vi "Core Action.vi"(8 "error in (no error)":errorcluster, 10 "SECS-II Class":refnum<class "SECS-II Class.lvclass">, 11 "24-Host Accepts On-Line Request from Equipment in":refnum<class "24-Host Accepts On-Line Request from Equipment.lvclass">) -> (0 "error out":errorcluster, 2 "SECS-II Class Out":refnum<class "SECS-II Class.lvclass">, 3 "24-Host Accepts On-Line Request from Equipment out":refnum<class "24-Host Accepts On-Line Request from Equipment.lvclass">)   [LabVIEW 2020, in "SECS Scenarios.lvlib" / "24-Host Accepts On-Line Request from Equipment.lvclass"]
uses:
  24-Host Accepts On-Line Request from Equipment.lvclass
  D:/Dropbox/SECS/SECS_GEM v1.1.0/Com/SECS Scenarios/Scenarios Class/Scenarios Class.lvclass
  SECS Communication/SECS-II Class/SECS-II Class.lvclass
  24-Host Accepts On-Line Request from Equipment.lvclass/24-Host Accepts On-Line Request from Equipment.ctl
  SECS Communication/S1 Message Class/S1 Message Class.lvclass
  D:/Dropbox/SECS/SECS_GEM v1.1.0/Com/SECS Communication/SECS-II Class/SECS-II Class.lvclass
  Scenarios Class/Scenarios Class.lvclass/Scenarios Class.ctl
  SECS Communication/SECS-II Class/SECS-II Class.lvclass/SECS-II Class.ctl
  Scenarios Class/Reply State.ctl
  SECS Communication/SECS-II Class/Read Function.vi
  Scenarios Class/Write Reply State.vi
  Scenarios Class/Read HSMS Class.vi
  SECS Communication/HSMS Class/HSMS Class.lvclass
  Scenarios Class/Scenarios Class.lvclass
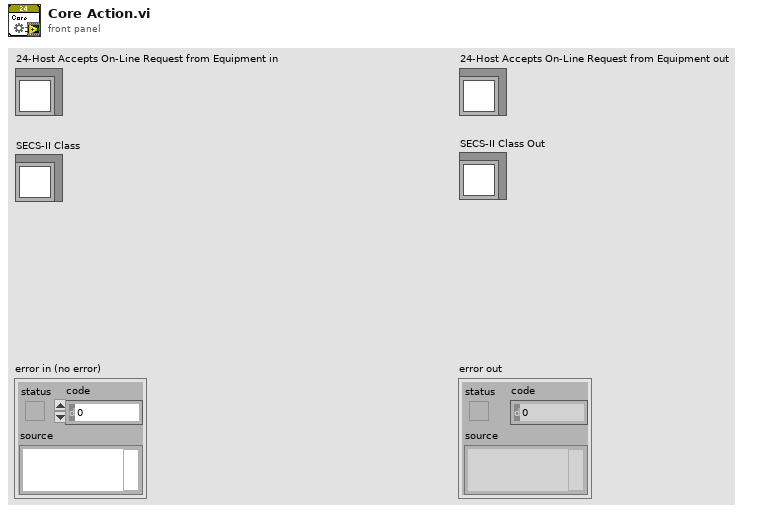
[diagram p1: front panel]
types:
  T1 = typedef "SECS Scenarios.lvlib/Scenarios Class.lvclass/Reply State.ctl" = enum16{"OK", "Illegal Data", "Unknown Stream", "Unknown Function", "Off-Line", "T3 Timeout", "Inner-Timeout"}
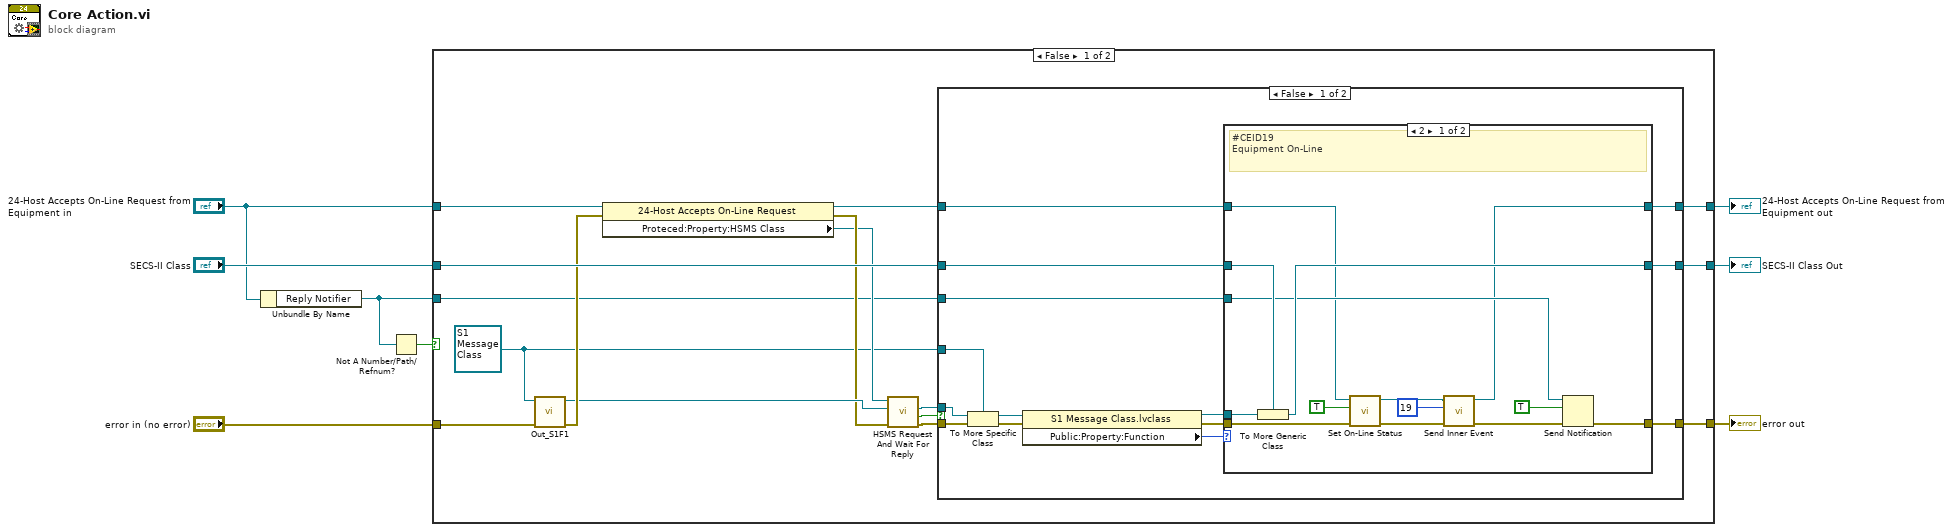
[diagram p0: block diagram]
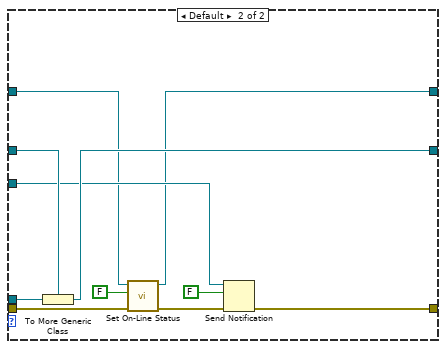
[diagram p2: hidden frame]
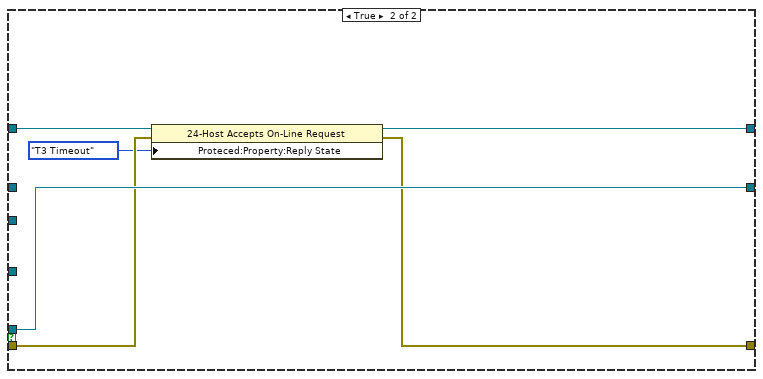
[diagram p3: hidden frame]
diagram:
  n1 = Unbundle By Name("24-Host Accepts On-Line Request from Equipment in") -> ("Reply Notifier"=w2:refnum<notifier>)
  n2 = Not A Number/Path/Refnum?(number/path/refnum=w2) -> (NaN/Path/Refnum?=w1:bool)
  n3 = case shown="False" w1 {
    tunnel: "error in (no error)" -> [w24 w72]
    tunnel: [w23 w70] -> w7
    tunnel: [w22 w72] -> w6
    tunnel: "SECS-II Class" -> [w21 w71]
    tunnel: [w20 w71] -> w4
    tunnel: "24-Host Accepts On-Line Request from Equipment in" -> [w10 w70]
    tunnel: w2 -> [w9 _]
    frame False {
      w11 = refnum<class "S1 Message Class.lvclass"> refnum ("S1 Message Class in")
      n4 = call "Out_S1F1.vi"("error in (no error)"=w24, "S1 Message Class in"=w11) -> ("error out"=w19:errorcluster, "S1 Message Class out"=w18:refnum<class "S1 Message Class.lvclass">)  [unwired: 8 in]
      n5 = property class="24-Host Accepts On-Line Request"(reference=w10, error in=w19) -> (reference out=w15:refnum<class "24-Host Accepts On-Line Request from Equipment.lvclass">, error out=w17:errorcluster, "Proteced:Property:HSMS Class"=w16:refnum<class "HSMS Class.lvclass">)
      n6 = call "HSMS Request And Wait For Reply.vi"("error in (no error)"=w17, "SECS-II Class In"=w18, "HSMS Class in"=w16) -> ("error out"=w12:errorcluster, "Timeout?"=w14:bool, "SECS-II Class Out"=w13:refnum<class "SECS-II Class.lvclass">)  [unwired: 5 in, 1 out]
      n7 = case shown="False" w14 {
        tunnel: w15 -> [w28 w68]
        tunnel: w13 -> [w37 w69]
        tunnel: w12 -> [w38 w67]
        tunnel: w11 -> [w36 _]
        tunnel: [w26 w65] -> w23
        tunnel: [w35 w64] -> w22
        tunnel: w21 -> [w30 _]
        tunnel: [w29 w69] -> w20
        tunnel: w9 -> [w25 _]
        frame False {
          n8 = To More Specific Class(target class=w36, reference=w37, error in=w38) -> (specific class reference=w33:refnum<class "S1 Message Class.lvclass">, error out=w34:errorcluster)
          n9 = property class="S1 Message Class.lvclass"(reference=w33, error in=w34) -> (reference out=w27:refnum<class "S1 Message Class.lvclass">, error out=w31:errorcluster, "Public:Property:Function"=w32:u8)
          n10 = case shown="2" w32 {
            tunnel: [w48 w59] -> w35
            tunnel: w31 -> [w46 w57]
            tunnel: w30 -> [w51 w62]
            tunnel: [w50 w61] -> w29
            tunnel: w28 -> [w45 w56]
            tunnel: w27 -> [w52 w63]
            tunnel: [w40 w54] -> w26
            tunnel: w25 -> [w47 w58]
            frame 2 {
              # "#CEID19\nEquipment On-Line"
              n11 = To More Generic Class(target class=w51, reference=w52) -> (generic class reference=w50:refnum<class "SECS-II Class.lvclass">)
              n12 = call "Set On-Line Status.vi"("error in (no error)"=w46, "On-Line"=TRUE, "Scenarios Class in"=w45) -> ("error out"=w43:errorcluster, "Scenarios Class out"=w41:refnum<class "24-Host Accepts On-Line Request from Equipment.lvclass">)  [unwired: 7 in]
              n13 = call "Send Inner Event.vi"("error in (no error)"=w43, "CEID"=u32 19, "Scenarios Class in"=w41) -> ("error out"=w39:errorcluster, "Scenarios Class out"=w40:refnum<class "24-Host Accepts On-Line Request from Equipment.lvclass">)  [unwired: 7 in]
              n14 = Send Notification(notification=TRUE, notifier=w47, error in (no error)=w39) -> (error out=w48:errorcluster)  [unwired: 1 out]
            }
            frame Default {
              n15 = To More Generic Class(target class=w62, reference=w63) -> (generic class reference=w61:refnum<class "SECS-II Class.lvclass">)
              n16 = call "Set On-Line Status.vi"("error in (no error)"=w57, "On-Line"=FALSE, "Scenarios Class in"=w56) -> ("error out"=w53:errorcluster, "Scenarios Class out"=w54:refnum<class "24-Host Accepts On-Line Request from Equipment.lvclass">)  [unwired: 7 in]
              n17 = Send Notification(notification=FALSE, notifier=w58, error in (no error)=w53) -> (error out=w59:errorcluster)  [unwired: 1 out]
            }
          }
        }
        frame True {
          n18 = property class="24-Host Accepts On-Line Request"(reference=w68, error in=w67, "Proteced:Property:Reply State"=Reply_State."T3 Timeout" ("Reply State")) -> (reference out=w65:refnum<class "24-Host Accepts On-Line Request from Equipment.lvclass">, error out=w64:errorcluster)
        }
      }
    }
    frame True {
    }
  }
  "error out" <- w6
  "24-Host Accepts On-Line Request from Equipment out" <- w7
  "SECS-II Class Out" <- w4
